vi "Convert Watt to dBm.vi"(4 "Watts":dbl format="%.2f") -> (1 "dBm":dbl format="%.2f")   [LabVIEW 2011]
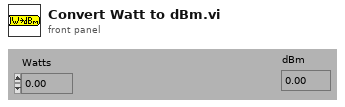
[diagram p1: front panel]
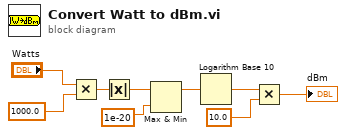
[diagram p0: block diagram]
diagram:
  n1 = Multiply(x="Watts", y=1000.0) -> (x*y=w8:dbl)
  n2 = Absolute Value(x=w8) -> (abs(x)=w3:dbl)
  n3 = Max & Min(x=w3, y=1e-20) -> (max(x,y)=w1:dbl)  [unwired: 1 out]
  n4 = Logarithm Base 10(1:w1) -> (0:w7:dbl)
  n5 = Multiply(x=w7, y=10.0) -> (x*y=→"dBm":dbl)
